vi "Read Timing Action Type.vi"(8 "error in (no error)":errorcluster, 11 "Timing Action in":refnum<class "Timing Action.lvclass">) -> (0 "error out":errorcluster, 2 "Timing Action Type":T1, 3 "Timing Action out":refnum<class "Timing Action.lvclass">)   [LabVIEW 2020, in "MacroAssert.lvlib" / "Timing Action.lvclass"]
uses:
  Timing Action.lvclass
  Timing Action Type.ctl
  Timing Action.lvclass/Timing Action.ctl
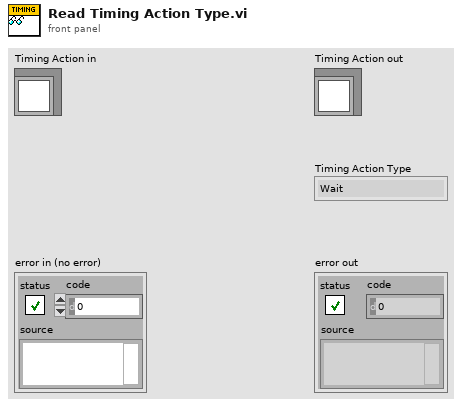
[diagram p1: front panel]
types:
  T1 = typedef "MacroAssert.lvlib/Timing Action.lvclass/Timing Action Type.ctl" = enum16{"Wait", "Wait Until"}
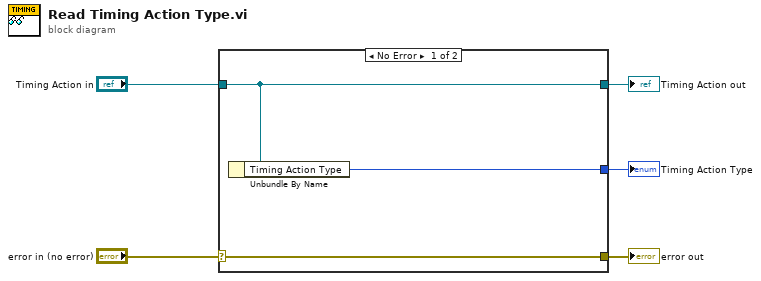
[diagram p0: block diagram]
diagram:
  n1 = case shown="No Error" "error in (no error)" {
    selector: "error in (no error)" -> [w8 w9]
    tunnel: [w8 w9] -> w4
    tunnel: [w7 w10] -> w2
    tunnel: "Timing Action in" -> [w7 w10]
    tunnel: [w6 _] -> w1
    frame No Error {
      n2 = Unbundle By Name(w7) -> ("Timing Action Type"=w6:T1)
    }
    frame Error {
    }
  }
  "error out" <- w4
  "Timing Action out" <- w2
  "Timing Action Type" <- w1
